vi "GetCollapsed.vi"(0 "reference in":refnum<class "PackageNode.lvclass">, 5 "error in (no error)":errorcluster) -> (14 "reference out":refnum<class "PackageNode.lvclass">, 15 "Collapsed":bool, 19 "error out":errorcluster)   [LabVIEW 2014, in "PackageNode.lvclass"]
uses:
  <resource>/Framework/Providers/Open_GDS/UML/PackageNode_class/PackageNode.lvclass
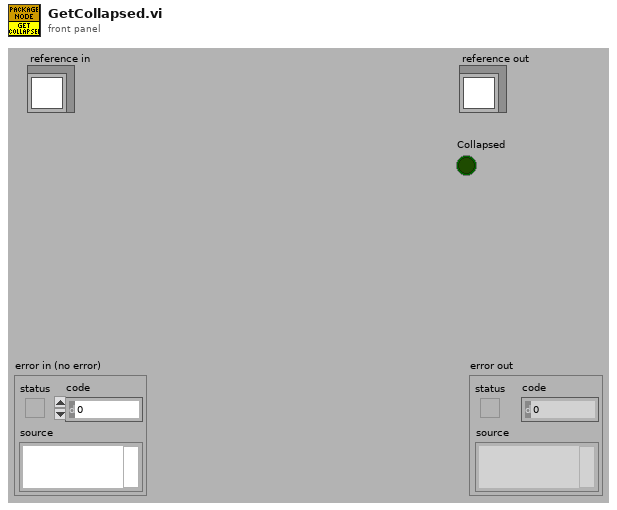
[diagram p1: front panel]
types:
  T1 = typedef "PackageNode.lvclass/ObjectAttributes.ctl" = cluster{"Base class":T2, "name":string, "contents":refnum<class "MultiLineString.lvclass">, "DEFAULT_TOP_WIDTH":i32, "DEFAULT_TOP_HEIGHT":i32, "DEFAULT_WIDTH":i32, "DEFAULT_HEIGHT":i32, "NAME_GAP":i32, "XGAP":i32, "YGAP":i32, "Collapsed":bool, "Note color":u32, "Justification":u16}
  T2 = typedef "RectangularNode.lvclass/ObjectAttributes.ctl" = cluster{"Base class":T3, "bounds":T4}
  T3 = typedef "AbstractNode.lvclass/ObjectAttributes.ctl" = cluster{"parent":refnum<class "AbstractNode.lvclass">, "children":refnum<class "AbstractNode.lvclass">[], "Hidden":bool}
  T4 = typedef "Rectangle Rectangle2D.ctl" = cluster{"x":dbl, "y":dbl, "width":dbl, "height":dbl}
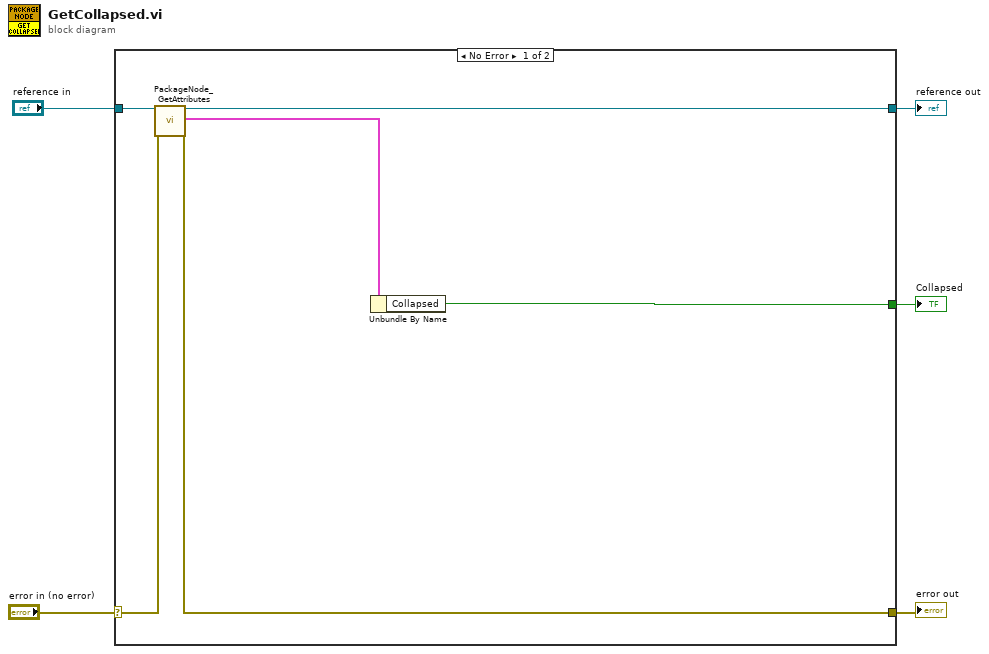
[diagram p0: block diagram]
diagram:
  n1 = case shown="No Error" "error in (no error)" {
    selector: "error in (no error)" -> [w11 w13]
    tunnel: [w9 w13] -> w4
    tunnel: [w7 w12] -> w2
    tunnel: "reference in" -> [w8 w12]
    tunnel: [w6 _] -> w1
    frame No Error {
      n2 = call <resource>:"PackageNode_GetAttributes.vi"("reference in"=w8, "error in (no error)"=w11) -> ("reference out"=w7:refnum<class "PackageNode.lvclass">, "Attributes"=w10:T1, "error out"=w9:errorcluster)  [unwired: 14 in, 1 out]
      n3 = Unbundle By Name(w10) -> ("Collapsed"=w6:bool)
    }
    frame Error {
    }
  }
  "error out" <- w4
  "reference out" <- w2
  "Collapsed" <- w1
